vi "Sync - Get All Sessions.vi"(0 "TSM context":T1, 11 "error in":errorcluster) -> (4 "TSM context out":T1, 6 "Sync Sessions Out":refnum<k15>[](array[refnum]), 15 "error out":errorcluster)   [LabVIEW 2019]
doc: "Returns all NI-Scope sessions in the Semiconductor Module Context."
uses:
  <vilib>/NI_TestStand_SemiconductorModule/NI_TestStand_Semiconductor_Module.lvlibp/PinMap/General/SemiconductorModuleContext.ctl
  <vilib>/NI_TestStand_SemiconductorModule/NI_TestStand_Semiconductor_Module.lvlibp
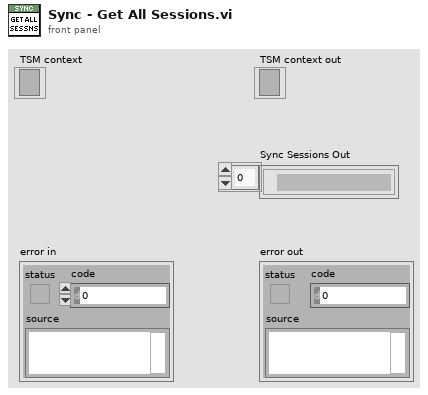
[diagram p1: front panel]
types:
  T1 = typedef "NI_TestStand_Semiconductor_Module.lvlibp/SemiconductorModuleContext.ctl" = refnum<k7>
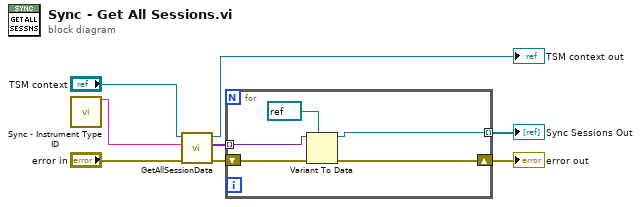
[diagram p0: block diagram]
diagram:
  n1 = call "Sync - Instrument Type ID.vi"() -> ("Instrument Type ID"=w2:string)  [unwired: 15 in]
  n2 = call <vilib>:"GetAllSessionData.vi"("error in (no error)"="error in", "Instrument Type Id"=w2, "Semiconductor Module Context"="TSM context") -> ("error out"=w5:errorcluster, "Session Data"=w4:variant[], "Semiconductor Module Context Out"=→"TSM context out":T1)  [unwired: 4 in, 2 out]
  n3 = for {
    tunnel: w4 -> [w12] mode=indexing
    tunnel: [w10] -> w1 mode=indexing
    shift-right: [w11] -> w3
    shift-left: w5 -> [w13]
    n4 = Variant To Data(error in=w13, type=refnum<k15> refnum ("instrument handle out"), Variant=w12) -> (data=w10:refnum<k15>, error out=w11:errorcluster)
  }
  "error out" <- w3
  "Sync Sessions Out" <- w1
